vi "FVI_manette_update global.vi"   [LabVIEW 2018]
uses:
  <vilib>/Rock Robotics/WPI/Utilities/WPI_GetSetVariantRefNum.vi
  MyGlobal.vi
  <vilib>/Rock Robotics/Network Tables/NT Write Numeric Array.vi
  <vilib>/Rock Robotics/Network Tables/NT Write Boolean Array.vi
types:
  T1 = typedef "WPI_JoystickDevRef.ctl" = cluster{"Device":T2}
  T2 = typedef "WPI_JoystickDeviceEnum.ctl" = enum16{"USB 0", "USB 1", "USB 2", "USB 3", "USB 4", "USB 5"}
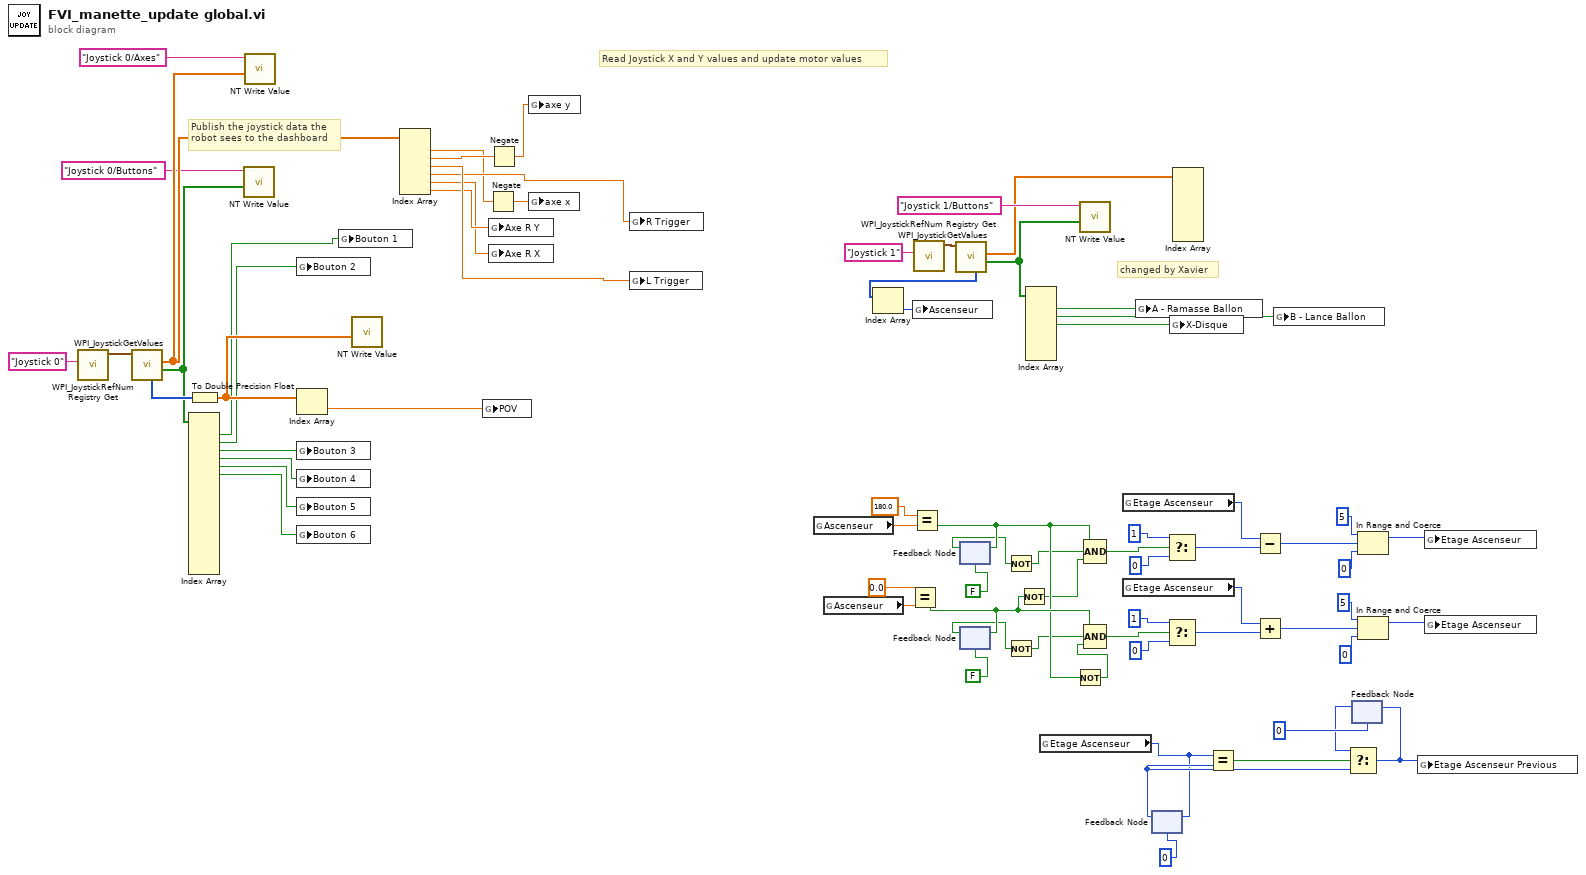
[diagram p0: block diagram]
diagram:
  # "changed by Xavier"
  # "Publish the joystick data the\nrobot sees to the dashboard"
  # "Read Joystick X and Y values and update motor values"
  n1 = call <vilib>:"WPI_JoystickRefNum Registry Get.vi"("refnum name"="Joystick 0") -> ("JoystickDevRef"=w3:T1)  [unwired: 1 in, 9 out]
  n2 = call <vilib>:"WPI_JoystickGetValues.vi"("JoystickDevRef"=w3) -> ("Buttons"=w7:bool[], "Axes"=w6:dbl[], "POVs"=w15:i16[])  [unwired: 6 in, 2 out]
  n3 = Index Array(array=w7) -> (element #1=w1:bool, element #2=w13:bool, element #3=w12:bool, element #4=w14:bool, element #5=w11:bool, element #6=w10:bool)  [unwired: 18 in, 12 out]
  n4 = To Double Precision Float(number=w15) -> (double precision float=w16:dbl[])
  n5 = call-poly <vilib>:"NT Write Value.vi"("Boolean Array"=w7, "Name"="Joystick 0/Buttons") -> ()  [unwired: 9 in, 1 out]
  n6 = call-poly <vilib>:"NT Write Value.vi"("Numeric Array"=w6, "Name"="Joystick 0/Axes") -> ()  [unwired: 9 in, 1 out]
  n7 = global write "MyGlobal.vi" "Bouton 2"(w13) -> ()
  n8 = Index Array(array=w16) -> (element=w72:dbl)  [unwired: 1 in]
  n9 = global write "MyGlobal.vi" "Bouton 3"(w12) -> ()
  n10 = global write "MyGlobal.vi" "Bouton 4"(w14) -> ()
  n11 = global write "MyGlobal.vi" "Bouton 5"(w11) -> ()
  n12 = global write "MyGlobal.vi" "Bouton 6"(w10) -> ()
  n13 = global write "MyGlobal.vi" "Bouton 1"(w1) -> ()
  n14 = call-poly <vilib>:"NT Write Value.vi"("Numeric Array"=w16) -> ()  [unwired: 10 in, 1 out]
  n15 = Index Array(array=w6) -> (element #1=w8:dbl, element #2=w9:dbl, element #3=w71:dbl, element #4=w70:dbl, element #5=w49:dbl, element #6=w50:dbl)  [unwired: 6 in]
  n16 = global write "MyGlobal.vi" "POV"(w72) -> ()
  n17 = Negate(x=w8) -> (-x=w47:dbl)
  n18 = Negate(x=w9) -> (-x=w48:dbl)
  n19 = global write "MyGlobal.vi" "Axe R Y"(w50) -> ()
  n20 = global write "MyGlobal.vi" "Axe R X"(w49) -> ()
  n21 = global write "MyGlobal.vi" "axe y"(w48) -> ()
  n22 = global write "MyGlobal.vi" "axe x"(w47) -> ()
  n23 = global write "MyGlobal.vi" "R Trigger"(w70) -> ()
  n24 = global write "MyGlobal.vi" "L Trigger"(w71) -> ()
  n25 = global read "MyGlobal.vi" "Ascenseur"() -> (w54:dbl)
  n26 = global read "MyGlobal.vi" "Ascenseur"() -> (w52:dbl)
  n27 = Equal?(x=0.0, y=w52) -> (x = y?=w68:bool)
  n28 = Equal?(x=180.0, y=w54) -> (x = y?=w66:bool)
  n29 = call <vilib>:"WPI_JoystickRefNum Registry Get.vi"("refnum name"="Joystick 1") -> ("JoystickDevRef"=w21:T1)  [unwired: 1 in, 9 out]
  n30 = call <vilib>:"WPI_JoystickGetValues.vi"("JoystickDevRef"=w21) -> ("Buttons"=w18:bool[], "Axes"=w19:dbl[], "POVs"=w64:i16[])  [unwired: 6 in, 2 out]
  n31 = Index Array(array=w64) -> (element=w65:i16)  [unwired: 1 in]
  n32 = global write "MyGlobal.vi" "Ascenseur"(w65) -> ()
  n33 = feedback #1(FALSE) -> (w25:bool)
  n34 = feedback-in #1(w66) -> ()
  n35 = feedback #2(FALSE) -> (w44:bool)
  n36 = feedback-in #2(w68) -> ()
  n37 = Not(x=w25) -> (.not. x?=w51:bool)
  n38 = Not(x=w44) -> (.not. x?=w45:bool)
  n39 = Not(x=w68) -> (.not. x?=w53:bool)
  n40 = Index Array(array=w18) -> (element #1=w23:bool, element #2=w17:bool, element #3=w63:bool)  [unwired: 7 in, 4 out]
  n41 = global read "MyGlobal.vi" "Etage Ascenseur"() -> (w56:u8)
  n42 = Not(x=w66) -> (.not. x?=w55:bool)
  n43 = call-poly <vilib>:"NT Write Value.vi"("Boolean Array"=w18, "Name"="Joystick 1/Buttons") -> ()  [unwired: 9 in, 1 out]
  n44 = Compound Arithmetic op=AND(w66, w51, w53) -> (w26:bool)
  n45 = Compound Arithmetic op=AND(w68, w45, w55) -> (w43:bool)
  n46 = global read "MyGlobal.vi" "Etage Ascenseur"() -> (w30:u8)
  n47 = global read "MyGlobal.vi" "Etage Ascenseur"() -> (w39:u8)
  n48 = global write "MyGlobal.vi" "A - Ramasse Ballon"(w23) -> ()
  n49 = feedback #3(0) -> (w59:i32)
  n50 = feedback-in #3(w56) -> ()
  n51 = Select(t=1, s=w26, f=0) -> (s? t:f=w29:i32)
  n52 = Select(t=1, s=w43, f=0) -> (s? t:f=w40:i32)
  n53 = global write "MyGlobal.vi" "X-Disque"(w63) -> ()
  n54 = Index Array(array=w19) -> ()  [unwired: 7 in, 7 out]
  n55 = Equal?(x=w56, y=w59) -> (x = y?=w58:bool)
  n56 = Subtract(x=w30, y=w29) -> (x-y=w31:i32)
  n57 = Add(x=w39, y=w40) -> (x+y=w38:i32)
  n58 = global write "MyGlobal.vi" "B - Lance Ballon"(w17) -> ()
  n59 = feedback #4(0) -> (w61:i32)
  n60 = Select(t=w61, s=w58, f=w59) -> (s? t:f=w60:i32)
  n61 = feedback-in #4(w60) -> ()
  n62 = In Range and Coerce(upper limit=5, x=w31, lower limit=0) -> (coerced(x)=w34:i32)  [unwired: 1 out]
  n63 = In Range and Coerce(upper limit=5, x=w38, lower limit=0) -> (coerced(x)=w35:i32)  [unwired: 1 out]
  n64 = global write "MyGlobal.vi" "Etage Ascenseur Previous"(w60) -> ()
  n65 = global write "MyGlobal.vi" "Etage Ascenseur"(w34) -> ()
  n66 = global write "MyGlobal.vi" "Etage Ascenseur"(w35) -> ()
